vi "current_measurement.vi"() -> ()   [LabVIEW 2017]
uses:
  <vilib>/Analysis/NI_AALBase.lvlib
  <vilib>/Analysis/baseanly.llb/Mean (DBL).vi
  <vilib>/DAQmx/read.llb/DAQmx Read (Analog 1D DBL 1Chan NSamp).vi
  <vilib>/DAQmx/create/channels.llb/DAQmx Create Channel (AI-Voltage-Basic).vi
panel:
  out "1/x":dbl format="%#_6p"
  out "I":dbl format="%#_6p"
  out "C":dbl format="%#_6p"
  in  "Resistor":dbl format="%#_13g"
  out "rc":dbl
  out "mean":dbl format="%0.2f"
  in  "physical channels":tag
  out "Waveform Chart":dbl(graph)
  in  "Stop Button":bool
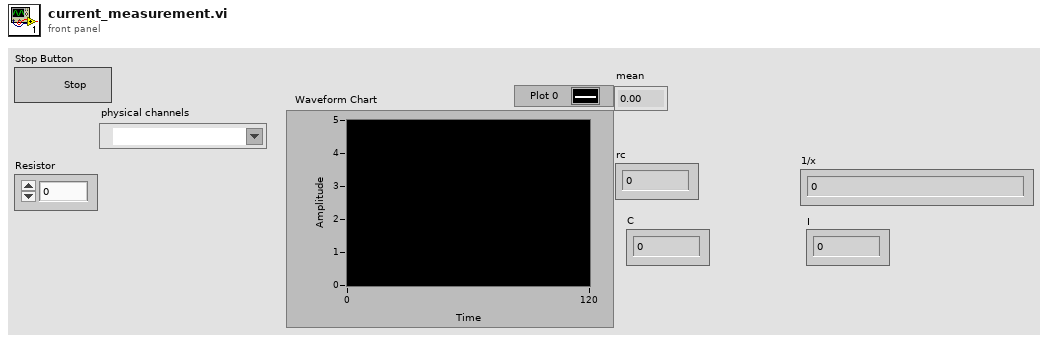
[diagram p1: front panel]
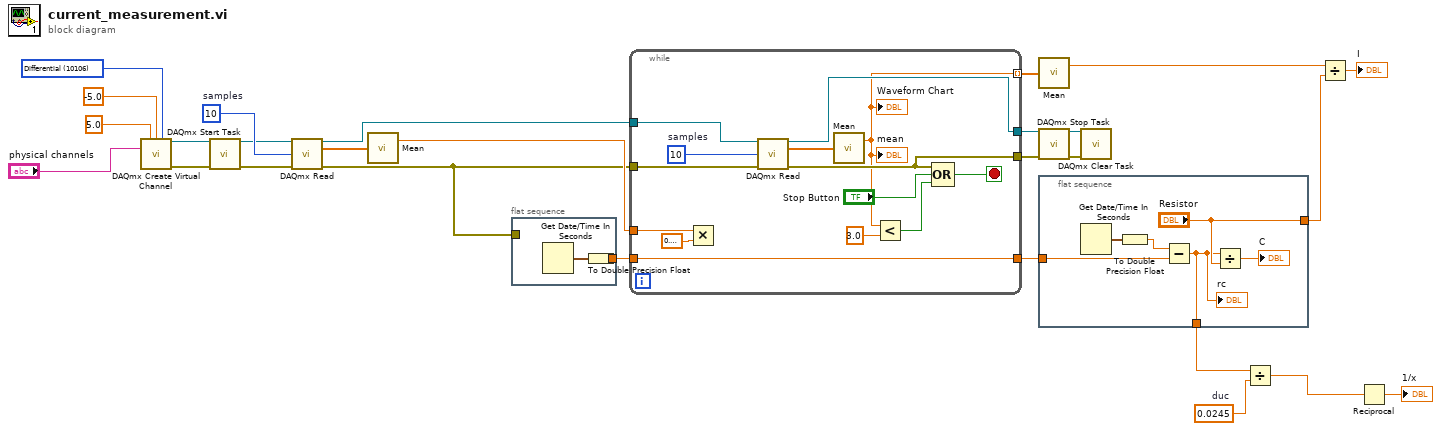
[diagram p0: block diagram]
diagram:
  w3 = 0.0245  # duc
  w14 = 10  # samples
  w20 = 10106 items=["Default"=-1, "RSE"=10083, "NRSE"=10078, "Differential"=10106, "Pseudodifferential"=12529] ("input terminal configuration")
  n1 = call-poly <vilib>:"DAQmx Create Virtual Channel.vi"("maximum value"=5.0, "minimum value"=-5.0, "input terminal configuration"=w20, "physical channels"="physical channels") -> ("task out"=w19:refnum<k21>, "error out"=w18:errorcluster)  [unwired: 10 in]
  n2 = call <vilib>:"DAQmx Start Task.vi"("task/channels in"=w19, "error in"=w18) -> ("task out"=w13:refnum<k21>, "error out"=w12:errorcluster)  [unwired: 12 in]
  n3 = call-poly <vilib>:"DAQmx Read.vi"("task/channels in"=w13, "number of samples per channel"=w14, "error in"=w12) -> ("task out"=w11:refnum<k21>, "data"=w15:dbl[], "error out"=w5:errorcluster)  [unwired: 10 in]
  n4 = call-poly <vilib>:"Mean.vi"("X"=w15) -> ("mean"=w10:dbl)  [unwired: 1 out]
  n5 = flat-sequence {
    tunnel: [w29] -> w17
    tunnel: w5 -> [_]
    frame #0 {
      n6 = Get Date/Time In Seconds() -> (seconds since 1Jan1904=w28:timestamp)
      n7 = To Double Precision Float(number=w28) -> (double precision float=w29:dbl)
    }
  }
  n8 = while {
    tunnel: [w40] -> w25
    tunnel: [w42] -> w24
    tunnel: w5 -> [w36]
    tunnel: w11 -> [w35]
    tunnel: w17 -> [w34]
    tunnel: [w34] -> w16
    tunnel: w10 -> [w33]
    tunnel: [w31] -> w9 mode=indexing
    stop <- w38 stop-if-true
    w43 = 10  # samples
    n9 = Multiply(x=w33, y=0.36787944117144233) -> ()  [unwired: 1 out]
    n10 = call-poly <vilib>:"DAQmx Read.vi"("task/channels in"=w35, "number of samples per channel"=w43, "error in"=w36) -> ("task out"=w42:refnum<k21>, "data"=w41:dbl[], "error out"=w40:errorcluster)  [unwired: 10 in]
    n11 = call-poly <vilib>:"Mean.vi"("X"=w41) -> ("mean"=w31:dbl)  [unwired: 1 out]
    "Waveform Chart" <- w31
    "mean" <- w31
    n12 = Less?(x=w31, y=3.0) -> (x < y?=w32:bool)
    n13 = Compound Arithmetic op=OR(w40, "Stop Button", w32) -> (w38:bool)
  }
  n14 = call-poly <vilib>:"Mean.vi"("X"=w9) -> ("mean"=w8:dbl)  [unwired: 1 out]
  n15 = call <vilib>:"DAQmx Stop Task.vi"("task/channels in"=w24, "error in"=w25) -> ("task out"=w26:refnum<k21>, "error out"=w27:errorcluster)  [unwired: 12 in]
  n16 = flat-sequence {
    tunnel: w16 -> [w47]
    tunnel: ["Resistor"] -> w7
    tunnel: [w44] -> w4
    frame #0 {
      n17 = Get Date/Time In Seconds() -> (seconds since 1Jan1904=w49:timestamp)
      n18 = To Double Precision Float(number=w49) -> (double precision float=w48:dbl)
      n19 = Subtract(x=w48, y=w47) -> (x-y=w44:dbl)
      "rc" <- w44
      n20 = Divide(x=w44, y="Resistor") -> (x/y=→"C":dbl)
    }
  }
  n21 = call <vilib>:"DAQmx Clear Task.vi"("task in"=w26, "error in"=w27) -> ()  [unwired: 13 in, 1 out]
  n22 = Divide(x=w4, y=w3) -> (x/y=w1:dbl)
  n23 = Divide(x=w8, y=w7) -> (x/y=→"I":dbl)
  n24 = Reciprocal(x=w1) -> (1/x=→"1/x":dbl)
